vi "EntoLidar_Octoplus.vi"() -> ()   [LabVIEW 2013, in "Octoplus_LIDAR.lvlib"]
uses:
  <userlib>/Octoplus_LIDAR/Octoplus_LIDAR.lvlib
  <vilib>/Analysis/baseanly.llb/Mean (DBL).vi
  <vilib>/Analysis/NI_AALBase.lvlib
  <vilib>/gmath/NI_Gmath.lvlib
panel:
  in  "Boolean":bool
  in  "End 2":dbl min=0.0 max=2047.0 step=1.0
  in  "Start 2":dbl min=0.0 max=2047.0 step=1.0
  out "Meter":dbl(knob) scale=0.0..10.0
  in  "Knob":dbl(knob) scale=0.0..10.0
  in  "End 1":dbl caption="End" min=0.0 max=2047.0 step=1.0
  in  "Start 1":dbl caption="Start" min=0.0 max=2047.0 step=1.0 format="%#_3f"
  in  "Tab Control":T1(tab)
  out "Signal":dbl[][](graph)
  out "Background":dbl[](graph)
  out "XY Graph 2":cluster{"X":dbl, "Y":dbl}[](graph)
  out "XY Graph 3":cluster{"X":dbl, "Y":dbl}[](graph)
  out "XY Graph 2":cluster{"X":dbl, "Y":dbl}[](graph)
  out "Air signal":cluster{timestamp[], dbl[]}(graph)
  out "XY Graph 4":cluster{"X":dbl, "Y":dbl}[](graph)
  in  "Buffer timesout (ms)":u32=30000
  in  "Nbr of lines in Image":u32=6000
  in  "File Path":path=path "C:/Users/USUARIO1/Desktop/Lidar test data"
  in  "Capture":bool
  in  "Record data":bool
  in  "Timeslot (cw, ts1, ts2)":i32(knob)=2 scale=0.0..2.0
  in  "start":bool
  in  "stop":bool
  in  "error in (no error)":errorcluster
  out "error out":errorcluster
  # "ROI 1"
  # "ROI 2"
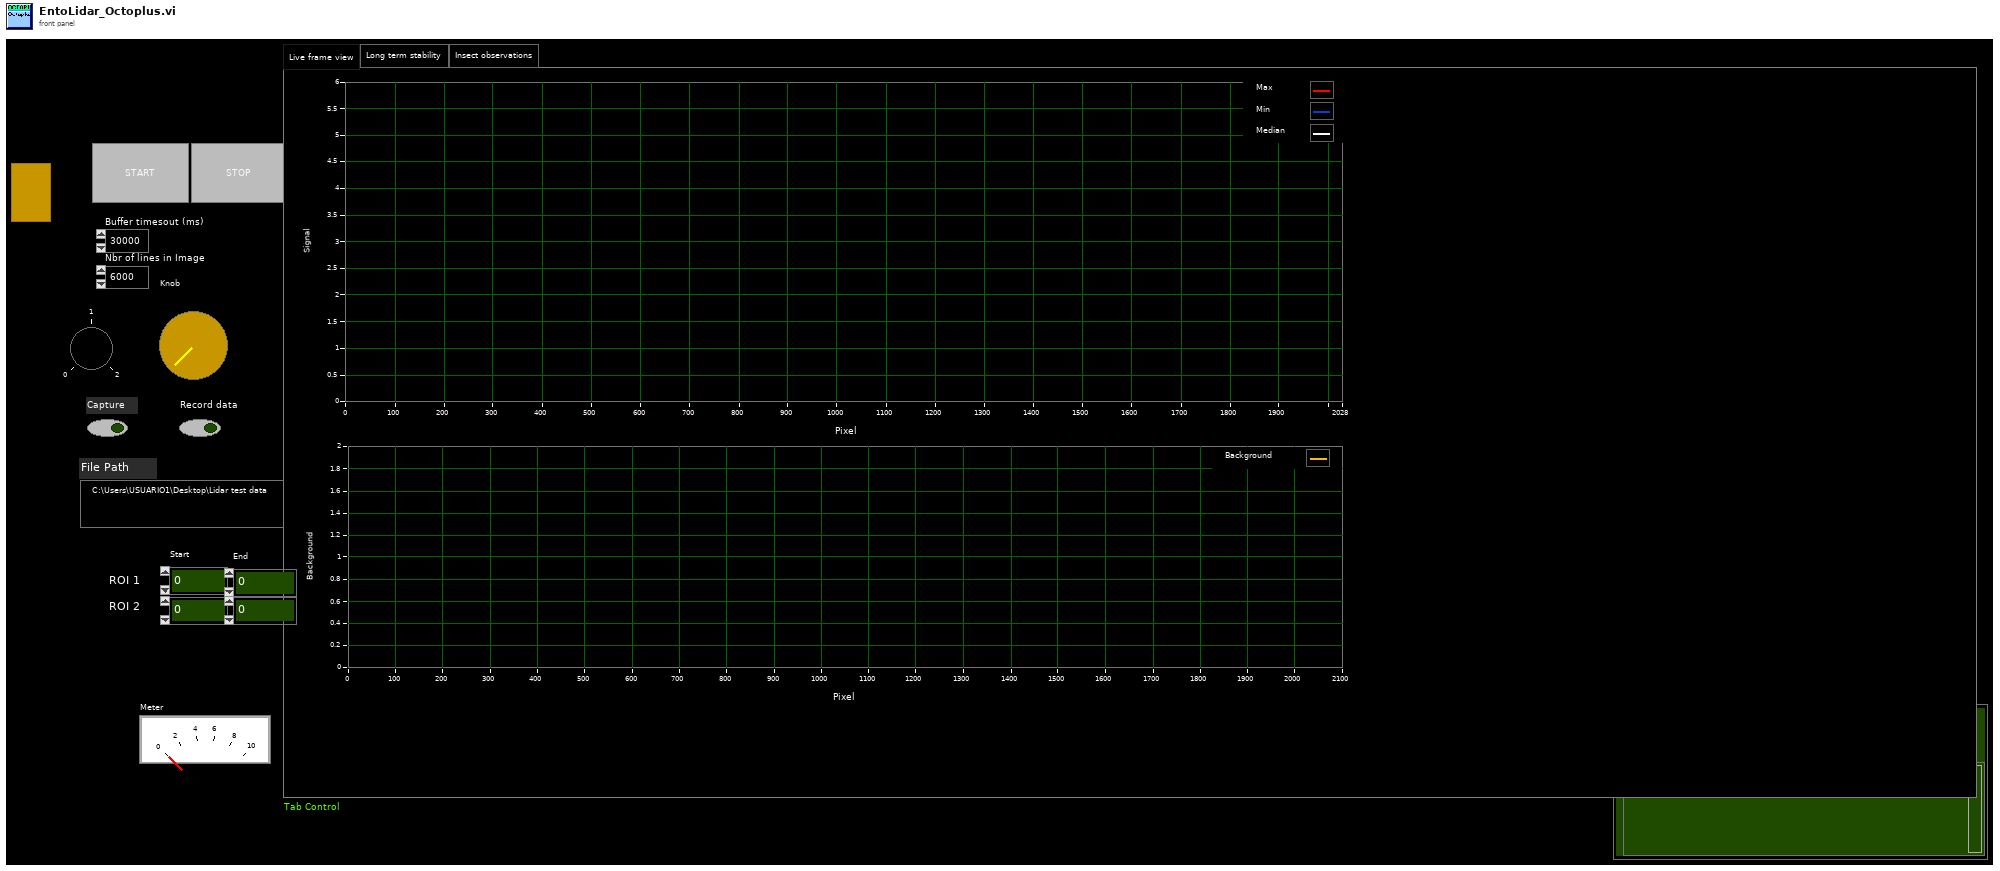
[diagram p1: front panel]
types:
  T1 = enum32{"Live frame view", "Long term stability", "Insect observations"}
  T2 = cluster{"pcID[0]":i8, "pcID[1]":i8, "pcID[2]":i8, "pcID[3]":i8, "pcID[4]":i8, "pcID[5]":i8, "pcID[6]":i8, "pcID[7]":i8, "pcID[8]":i8, "pcID[9]":i8, "pcID[10]":i8, "pcID[11]":i8, "pcID[12]":i8, "pcID[13]":i8, "pcID[14]":i8, "pcID[15]":i8, "pcID[16]":i8, "pcID[17]":i8, "pcID[18]":i8, "pcID[19]":i8, "pcID[20]":i8, "pcID[21]":i8, "pcID[22]":i8, "pcID[23]":i8, "pcID[24]":i8, "pcID[25]":i8, "pcID[26]":i8, "pcID[27]":i8, "pcID[28]":i8, "pcID[29]":i8, "pcID[30]":i8, "pcID[31]":i8, "pcID[32]":i8, "pcID[33]":i8, "pcID[34]":i8, "pcID[35]":i8, "pcID[36]":i8, "pcID[37]":i8, "pcID[38]":i8, "pcID[39]":i8, "pcID[40]":i8, "pcID[41]":i8, "pcID[42]":i8, "pcID[43]":i8, "pcID[44]":i8, "pcID[45]":i8, "pcID[46]":i8, "pcID[47]":i8, "pcID[48]":i8, "pcID[49]":i8, "pcID[50]":i8, "pcID[51]":i8, "pcID[52]":i8, "pcID[53]":i8, "pcID[54]":i8, "pcID[55]":i8, "pcID[56]":i8, "pcID[57]":i8, "pcID[58]":i8, "pcID[59]":i8, "pcID[60]":i8, "pcID[61]":i8, "pcID[62]":i8, "pcID[63]":i8, "pcID[64]":i8, "pcID[65]":i8, "pcID[66]":i8, "pcID[67]":i8, "pcID[68]":i8, "pcID[69]":i8, "pcID[70]":i8, "pcID[71]":i8, "pcID[72]":i8, "pcID[73]":i8, "pcID[74]":i8, "pcID[75]":i8, "pcID[76]":i8, "pcID[77]":i8, "pcID[78]":i8, "pcID[79]":i8, "pcID[80]":i8, "pcID[81]":i8, "pcID[82]":i8, "pcID[83]":i8, "pcID[84]":i8, "pcID[85]":i8, "pcID[86]":i8, "pcID[87]":i8, "pcID[88]":i8, "pcID[89]":i8, "pcID[90]":i8, "pcID[91]":i8, "pcID[92]":i8, "pcID[93]":i8, "pcID[94]":i8, "pcID[95]":i8, "pcID[96]":i8, "pcID[97]":i8, "pcID[98]":i8, "pcID[99]":i8, "pcID[100]":i8, "pcID[101]":i8, "pcID[102]":i8, "pcID[103]":i8, "pcID[104]":i8, "pcID[105]":i8, "pcID[106]":i8, "pcID[107]":i8, "pcID[108]":i8, "pcID[109]":i8, "pcID[110]":i8, "pcID[111]":i8, "pcID[112]":i8, "pcID[113]":i8, "pcID[114]":i8, "pcID[115]":i8, "pcID[116]":i8, "pcID[117]":i8, "pcID[118]":i8, "pcID[119]":i8, "pcID[120]":i8, "pcID[121]":i8, "pcID[122]":i8, "pcID[123]":i8, "pcID[124]":i8, "pcID[125]":i8, "pcID[126]":i8, "pcID[127]":i8, "pcID[128]":i8, "pcID[129]":i8, "pcID[130]":i8, "pcID[131]":i8, "pcID[132]":i8, "pcID[133]":i8, "pcID[134]":i8, "pcID[135]":i8, "pcID[136]":i8, "pcID[137]":i8, "pcID[138]":i8, "pcID[139]":i8, "pcID[140]":i8, "pcID[141]":i8, "pcID[142]":i8, "pcID[143]":i8, "pcID[144]":i8, "pcID[145]":i8, "pcID[146]":i8, "pcID[147]":i8, "pcID[148]":i8, "pcID[149]":i8, "pcID[150]":i8, "pcID[151]":i8, "pcID[152]":i8, "pcID[153]":i8, "pcID[154]":i8, "pcID[155]":i8, "pcID[156]":i8, "pcID[157]":i8, "pcID[158]":i8, "pcID[159]":i8, "pcID[160]":i8, "pcID[161]":i8, "pcID[162]":i8, "pcID[163]":i8, "pcID[164]":i8, "pcID[165]":i8, "pcID[166]":i8, "pcID[167]":i8, "pcID[168]":i8, "pcID[169]":i8, "pcID[170]":i8, "pcID[171]":i8, "pcID[172]":i8, "pcID[173]":i8, "pcID[174]":i8, "pcID[175]":i8, "pcID[176]":i8, "pcID[177]":i8, "pcID[178]":i8, "pcID[179]":i8, "pcID[180]":i8, "pcID[181]":i8, "pcID[182]":i8, "pcID[183]":i8, "pcID[184]":i8, "pcID[185]":i8, "pcID[186]":i8, "pcID[187]":i8, "pcID[188]":i8, "pcID[189]":i8, "pcID[190]":i8, "pcID[191]":i8, "pcID[192]":i8, "pcID[193]":i8, "pcID[194]":i8, "pcID[195]":i8, "pcID[196]":i8, "pcID[197]":i8, "pcID[198]":i8, "pcID[199]":i8, "pcID[200]":i8, "pcID[201]":i8, "pcID[202]":i8, "pcID[203]":i8, "pcID[204]":i8, "pcID[205]":i8, "pcID[206]":i8, "pcID[207]":i8, "pcID[208]":i8, "pcID[209]":i8, "pcID[210]":i8, "pcID[211]":i8, "pcID[212]":i8, "pcID[213]":i8, "pcID[214]":i8, "pcID[215]":i8, "pcID[216]":i8, "pcID[217]":i8, "pcID[218]":i8, "pcID[219]":i8, "pcID[220]":i8, "pcID[221]":i8, "pcID[222]":i8, "pcID[223]":i8, "pcID[224]":i8, "pcID[225]":i8, "pcID[226]":i8, "pcID[227]":i8, "pcID[228]":i8, "pcID[229]":i8, "pcID[230]":i8, "pcID[231]":i8, "pcID[232]":i8, "pcID[233]":i8, "pcID[234]":i8, "pcID[235]":i8, "pcID[236]":i8, "pcID[237]":i8, "pcID[238]":i8, "pcID[239]":i8, "pcID[240]":i8, "pcID[241]":i8, "pcID[242]":i8, "pcID[243]":i8, "pcID[244]":i8, "pcID[245]":i8, "pcID[246]":i8, "pcID[247]":i8, "pcID[248]":i8, "pcID[249]":i8, "pcID[250]":i8, "pcID[251]":i8, "pcID[252]":i8, "pcID[253]":i8, "pcID[254]":i8, "pcID[255]":i8, "pcID[256]":i8, "pcID[257]":i8, "pcID[258]":i8, "pcID[259]":i8}
  T3 = enum16{"open", "replace", "create", "open or create", "replace or create", "replace or create with confirmation"}
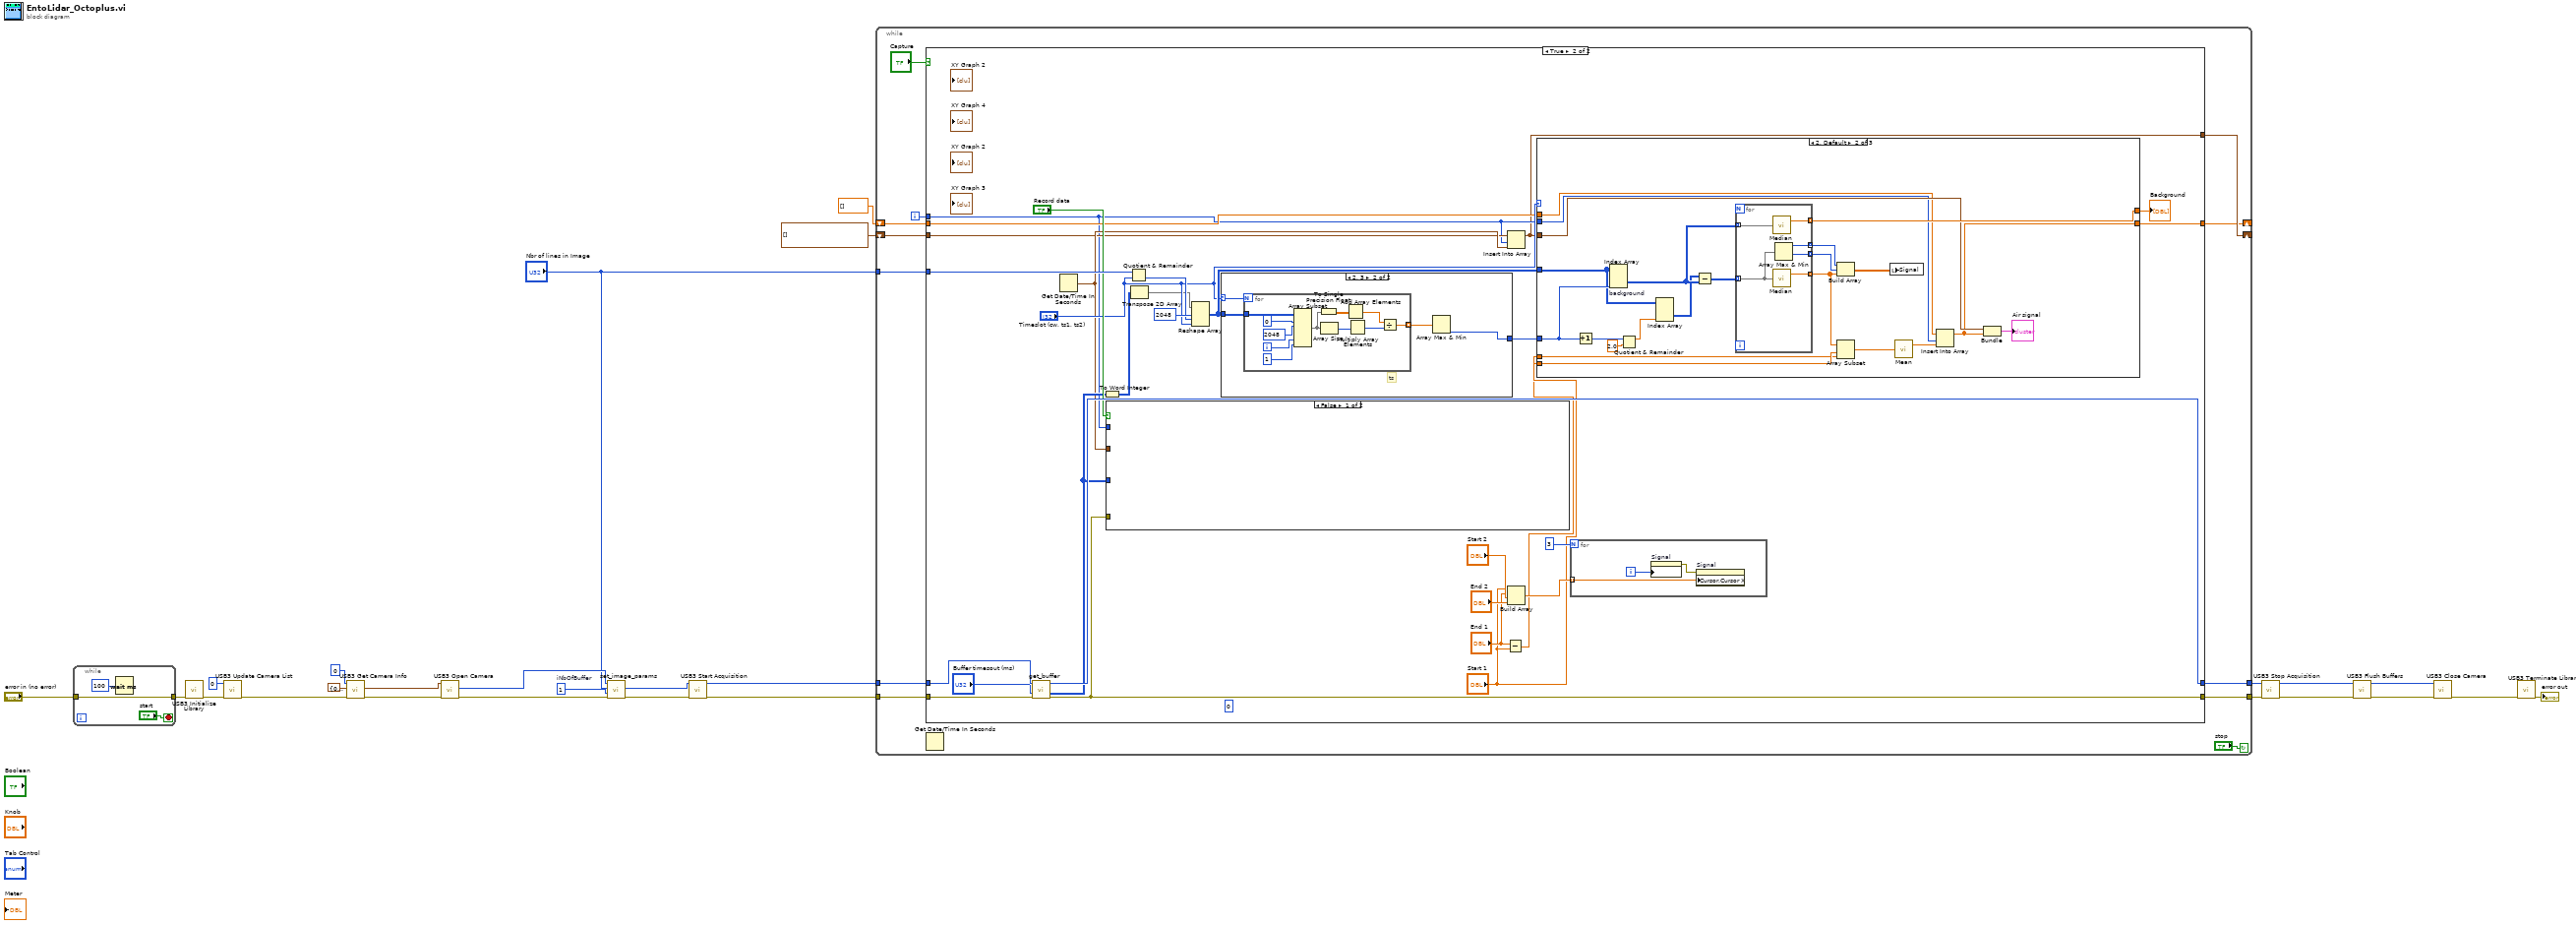
[diagram p0: block diagram]
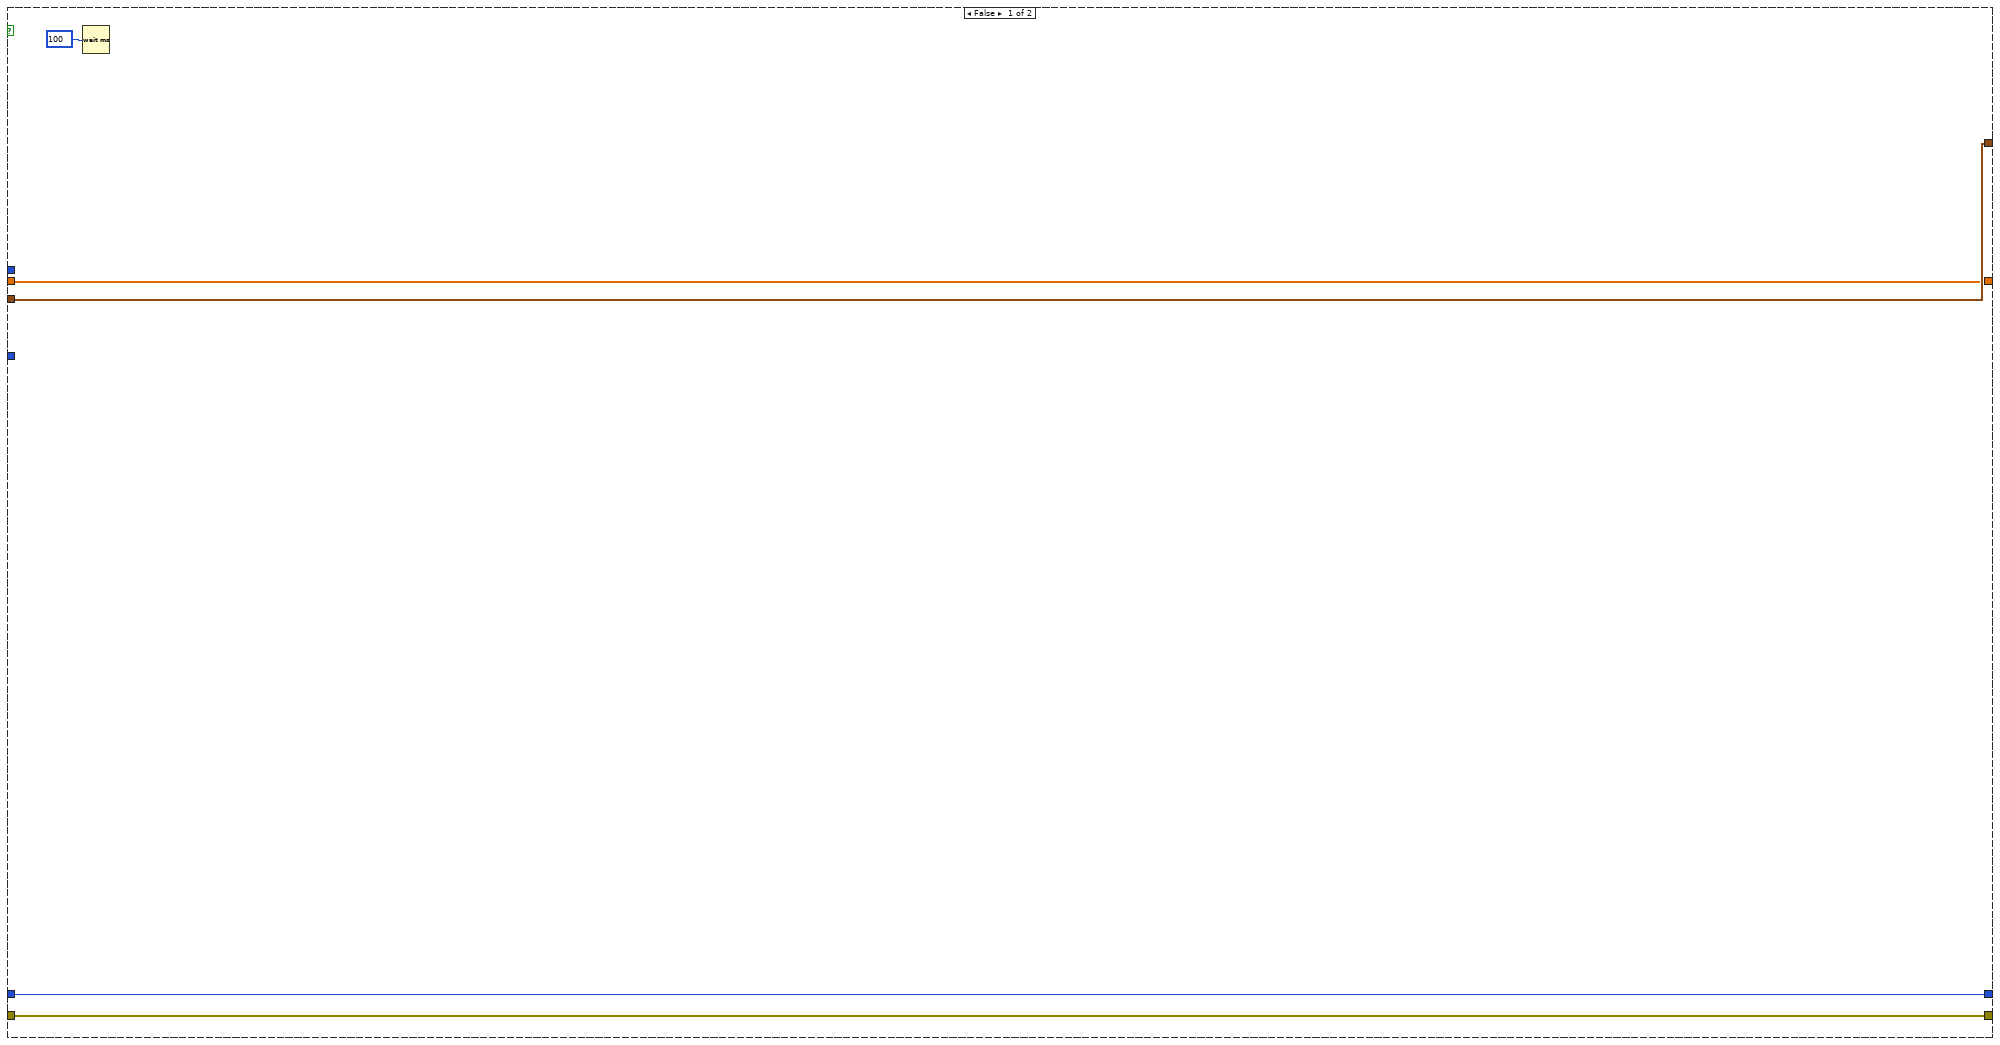
[diagram p2: hidden frame]
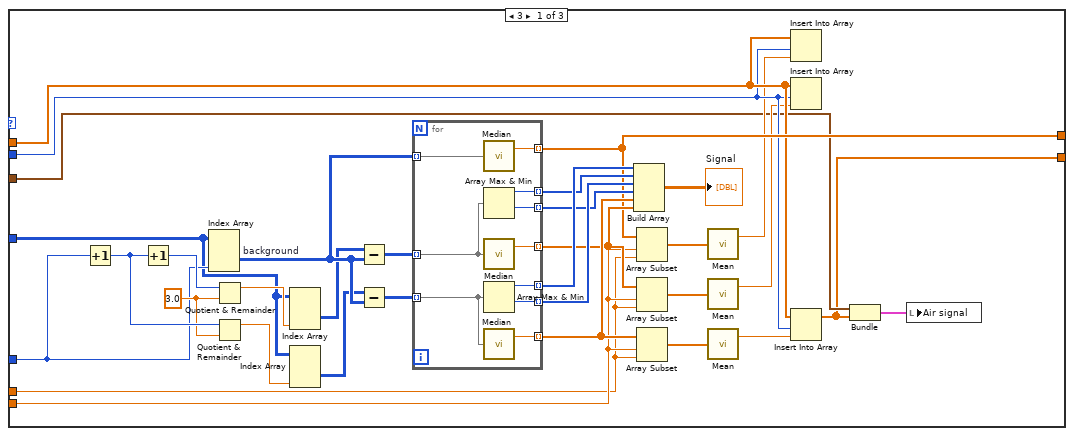
[diagram p3: hidden frame]
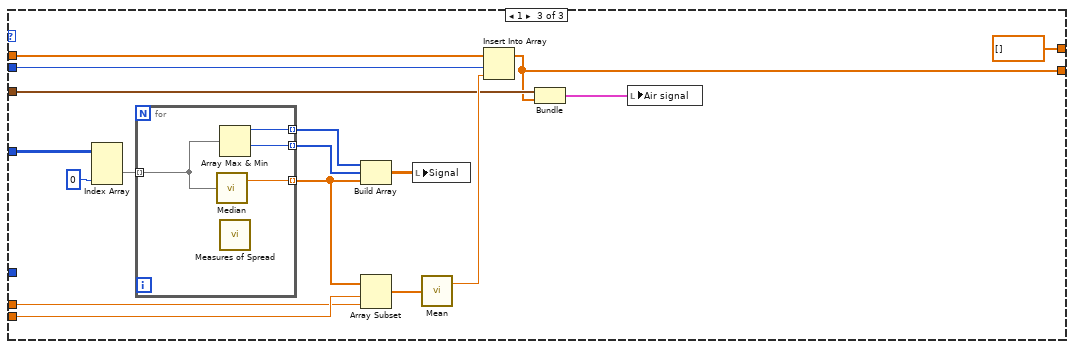
[diagram p4: hidden frame]
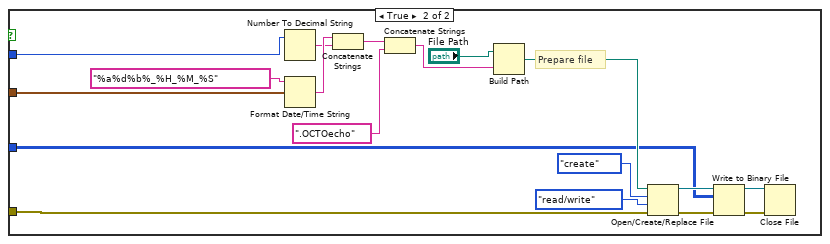
[diagram p5: hidden frame]
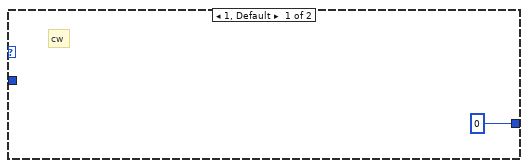
[diagram p6: hidden frame]
diagram:
  w19 = u32 1  # iNbOfBuffer
  n1 = while {
    tunnel: "error in (no error)" -> [w30]
    tunnel: [w30] -> w4
    stop <- "start" stop-if-true
    n2 = Wait (ms)(milliseconds to wait=u32 100) -> ()  [unwired: 1 out]
  }
  n3 = call <userlib>:"USB3 Initialize Library.vi"("error in (no error)"=w4) -> ("error out"=w6:errorcluster)  [unwired: 8 in, 1 out]
  n4 = call <userlib>:"USB3 Update Camera List.vi"("error in (no error)"=w6, "pulNbCameras"=u32 0) -> ("error out"=w24:errorcluster)  [unwired: 7 in, 2 out]
  n5 = call <userlib>:"USB3 Get Camera Info.vi"("error in (no error)"=w24, "pCameraInfo"=T2 {"pcID[0]"=0, "pcID[1]"=0, "pcID[2]"=0, "pcID[3]"=0, "pcID[4]"=0, "pcID[5]"=0, "pcID[6]"=0, "pcID[7]"=0, "pcID[8]"=0, "pcID[9]"=0, "pcID[10]"=0, "pcID[11]"=0, "pcID[12]"=0, "pcID[13]"=0, "pcID[14]"=0, "pcID[15]"=0, "pcID[16]"=0, "pcID[17]"=0, "pcID[18]"=0, "pcID[19]"=0, "pcID[20]"=0, "pcID[21]"=0, "pcID[22]"=0, "pcID[23]"=0, "pcID[24]"=0, "pcID[25]"=0, "pcID[26]"=0, "pcID[27]"=0, "pcID[28]"=0, "pcID[29]"=0, "pcID[30]"=0, "pcID[31]"=0, "pcID[32]"=0, "pcID[33]"=0, "pcID[34]"=0, "pcID[35]"=0, "pcID[36]"=0, "pcID[37]"=0, "pcID[38]"=0, "pcID[39]"=0, "pcID[40]"=0, "pcID[41]"=0, "pcID[42]"=0, "pcID[43]"=0, "pcID[44]"=0, "pcID[45]"=0, "pcID[46]"=0, "pcID[47]"=0, "pcID[48]"=0, "pcID[49]"=0, "pcID[50]"=0, "pcID[51]"=0, "pcID[52]"=0, "pcID[53]"=0, "pcID[54]"=0, "pcID[55]"=0, "pcID[56]"=0, "pcID[57]"=0, "pcID[58]"=0, "pcID[59]"=0, "pcID[60]"=0, "pcID[61]"=0, "pcID[62]"=0, "pcID[63]"=0, "pcID[64]"=0, "pcID[65]"=0, "pcID[66]"=0, "pcID[67]"=0, "pcID[68]"=0, "pcID[69]"=0, "pcID[70]"=0, "pcID[71]"=0, "pcID[72]"=0, "pcID[73]"=0, "pcID[74]"=0, "pcID[75]"=0, "pcID[76]"=0, "pcID[77]"=0, "pcID[78]"=0, "pcID[79]"=0, "pcID[80]"=0, "pcID[81]"=0, "pcID[82]"=0, "pcID[83]"=0, "pcID[84]"=0, "pcID[85]"=0, "pcID[86]"=0, "pcID[87]"=0, "pcID[88]"=0, "pcID[89]"=0, "pcID[90]"=0, "pcID[91]"=0, "pcID[92]"=0, "pcID[93]"=0, "pcID[94]"=0, "pcID[95]"=0, "pcID[96]"=0, "pcID[97]"=0, "pcID[98]"=0, "pcID[99]"=0, "pcID[100]"=0, "pcID[101]"=0, "pcID[102]"=0, "pcID[103]"=0, "pcID[104]"=0, "pcID[105]"=0, "pcID[106]"=0, "pcID[107]"=0, "pcID[108]"=0, "pcID[109]"=0, "pcID[110]"=0, "pcID[111]"=0, "pcID[112]"=0, "pcID[113]"=0, "pcID[114]"=0, "pcID[115]"=0, "pcID[116]"=0, "pcID[117]"=0, "pcID[118]"=0, "pcID[119]"=0, "pcID[120]"=0, "pcID[121]"=0, "pcID[122]"=0, "pcID[123]"=0, "pcID[124]"=0, "pcID[125]"=0, "pcID[126]"=0, "pcID[127]"=0, "pcID[128]"=0, "pcID[129]"=0, "pcID[130]"=0, "pcID[131]"=0, "pcID[132]"=0, "pcID[133]"=0, "pcID[134]"=0, "pcID[135]"=0, "pcID[136]"=0, "pcID[137]"=0, "pcID[138]"=0, "pcID[139]"=0, "pcID[140]"=0, "pcID[141]"=0, "pcID[142]"=0, "pcID[143]"=0, "pcID[144]"=0, "pcID[145]"=0, "pcID[146]"=0, "pcID[147]"=0, "pcID[148]"=0, "pcID[149]"=0, "pcID[150]"=0, "pcID[151]"=0, "pcID[152]"=0, "pcID[153]"=0, "pcID[154]"=0, "pcID[155]"=0, "pcID[156]"=0, "pcID[157]"=0, "pcID[158]"=0, "pcID[159]"=0, "pcID[160]"=0, "pcID[161]"=0, "pcID[162]"=0, "pcID[163]"=0, "pcID[164]"=0, "pcID[165]"=0, "pcID[166]"=0, "pcID[167]"=0, "pcID[168]"=0, "pcID[169]"=0, "pcID[170]"=0, "pcID[171]"=0, "pcID[172]"=0, "pcID[173]"=0, "pcID[174]"=0, "pcID[175]"=0, "pcID[176]"=0, "pcID[177]"=0, "pcID[178]"=0, "pcID[179]"=0, "pcID[180]"=0, "pcID[181]"=0, "pcID[182]"=0, "pcID[183]"=0, "pcID[184]"=0, "pcID[185]"=0, "pcID[186]"=0, "pcID[187]"=0, "pcID[188]"=0, "pcID[189]"=0, "pcID[190]"=0, "pcID[191]"=0, "pcID[192]"=0, "pcID[193]"=0, "pcID[194]"=0, "pcID[195]"=0, "pcID[196]"=0, "pcID[197]"=0, "pcID[198]"=0, "pcID[199]"=0, "pcID[200]"=0, "pcID[201]"=0, "pcID[202]"=0, "pcID[203]"=0, "pcID[204]"=0, "pcID[205]"=0, "pcID[206]"=0, "pcID[207]"=0, "pcID[208]"=0, "pcID[209]"=0, "pcID[210]"=0, "pcID[211]"=0, "pcID[212]"=0, "pcID[213]"=0, "pcID[214]"=0, "pcID[215]"=0, "pcID[216]"=0, "pcID[217]"=0, "pcID[218]"=0, "pcID[219]"=0, "pcID[220]"=0, "pcID[221]"=0, "pcID[222]"=0, "pcID[223]"=0, "pcID[224]"=0, "pcID[225]"=0, "pcID[226]"=0, "pcID[227]"=0, "pcID[228]"=0, "pcID[229]"=0, "pcID[230]"=0, "pcID[231]"=0, "pcID[232]"=0, "pcID[233]"=0, "pcID[234]"=0, "pcID[235]"=0, "pcID[236]"=0, "pcID[237]"=0, "pcID[238]"=0, "pcID[239]"=0, "pcID[240]"=0, "pcID[241]"=0, "pcID[242]"=0, "pcID[243]"=0, "pcID[244]"=0, "pcID[245]"=0, "pcID[246]"=0, "pcID[247]"=0, "pcID[248]"=0, "pcID[249]"=0, "pcID[250]"=0, "pcID[251]"=0, "pcID[252]"=0, "pcID[253]"=0, "pcID[254]"=0, "pcID[255]"=0, "pcID[256]"=0, "pcID[257]"=0, "pcID[258]"=0, "pcID[259]"=0}, "ulIndex"=u32 0) -> ("error out"=w22:errorcluster, "pCameraInfo out"=w23:T2)  [unwired: 6 in, 1 out]
  n6 = call <userlib>:"USB3 Open Camera.vi"("error in (no error)"=w22, "pCameraInfo"=w23) -> ("error out"=w21:errorcluster, "hCamera"=w20:u64)  [unwired: 7 in, 1 out]
  n7 = call <userlib>:"set_image_params.vi"("error in (no error)"=w21, "iNbOfBuffer"=w19, "iImageHeight"="Nbr of lines in Image", "hCamera"=w20) -> ("error out"=w18:errorcluster, "hCamera"=w9:u64)  [unwired: 5 in, 1 out]
  n8 = call <userlib>:"USB3 Start Acquisition.vi"("error in (no error)"=w18, "hCamera"=w9) -> ("error out"=w16:errorcluster, "hCamera"=w17:u64)  [unwired: 7 in, 1 out]
  n9 = while {
    tunnel: w17 -> [w42]
    tunnel: w16 -> [w41]
    tunnel: [w38] -> w15
    tunnel: [w40] -> w12
    tunnel: "Nbr of lines in Image" -> [w36]
    shift-right: [w34] -> _
    shift-left: timestamp[] [] -> [w33]
    shift-right: [w32] -> _
    shift-left: dbl[] [] -> [w31]
    i -> [w35]
    stop <- "stop" continue-if-true
    n10 = case shown="True" "Capture" {
      tunnel: w42 -> [w45 w76]
      tunnel: w41 -> [w46 w75]
      tunnel: [w45 w74] -> w40
      tunnel: [w46 w67] -> w38
      tunnel: w36 -> [_ w70]
      tunnel: w35 -> [_ w50]
      tunnel: [w44 w49] -> w34
      tunnel: w33 -> [w44 w55]
      tunnel: w31 -> [w43 w51]
      tunnel: [w43 w48] -> w32
      frame False {
        n11 = Wait (ms)(milliseconds to wait=u32 100) -> ()  [unwired: 1 out]
      }
      frame True {
        (unwired) 0 ("index")
        n12 = call <userlib>:"get_buffer.vi"("error in (no error)"=w75, "ulTimeoutInMs"="Buffer timesout (ms)", "hCamera"=w76) -> ("error out"=w67:errorcluster, "output array"=w61:u16[][], "hCamera out"=w74:u64)  [unwired: 5 in, 1 out]
        n13 = Get Date/Time In Seconds() -> (seconds since 1Jan1904=w56:timestamp)
        n14 = To Word Integer(number=w61) -> (16bit integer=w62:i16[][])
        n15 = case shown="False" "Record data" {
          tunnel: w67 -> [_ w182]
          tunnel: w61 -> [_ w177]
          tunnel: w50 -> [_ w173]
          tunnel: w56 -> [_ w172]
          frame False {
          }
          frame True {
            # "Prepare file"
            n16 = Number To Decimal String(number=w173) -> (decimal integer string=w174:string)  [unwired: 1 in]
            n17 = Format Date/Time String(time format string (%c)="%a%d%b%_%H_%M_%S", seconds (now)=w172) -> (date/time string=w175:string)  [unwired: 1 in]
            n18 = Concatenate Strings(w175, w174) -> (w176:string)
            n19 = Concatenate Strings(w176, ".OCTOecho") -> (w179:string)
            n20 = Build Path(base path="File Path", name or relative path=w179) -> (appended path=w181:path)
            n21 = Open/Create/Replace File(file path (use dialog)=w181, error in=w182, operation (0:open)=T3."create", access (0:read/write)=enum16{"read/write", "read-only", "write-only"}."read/write") -> (refnum out=w187:refnum<file>, error out=w183:errorcluster)  [unwired: 3 out]
            n22 = Write to Binary File(file (use dialog)=w187, data=w177, error in=w183) -> (refnum out=w185:refnum<file>, error out=w184:errorcluster)  [unwired: 1 in, 3 out]
            n23 = Close File(refnum=w185, error in=w184) -> ()  [unwired: 2 out]
          }
        }
        n24 = Quotient & Remainder(x=w70, y="Timeslot (cw, ts1, ts2)") -> (floor(x/y)=w69:u32)  [unwired: 1 out]
        n25 = Transpose 2D Array(2D array=w62) -> (transposed array=w63:i16[][])
        n26 = Reshape Array(w63, 2048 ("dimension size"), w69, "Timeslot (cw, ts1, ts2)") -> (w65:i16[][][])
        n27 = case shown="2, 3" "Timeslot (cw, ts1, ts2)" {
          selector: "Timeslot (cw, ts1, ts2)" -> [_ w191]
          tunnel: [0 w193] -> w66
          tunnel: w65 -> [_ w192]
          frame 1, Default {
            # "cw"
          }
          frame 2, 3 {
            # "ts"
            n28 = for {
              N: w191 -> [_]
              tunnel: [w204] -> w194 mode=indexing
              tunnel: w192 -> [w199]
              i -> [w201]
              n29 = Array Subset(array=w199, index (dim 0)=0 ("index"), length (dim 0)=2048 ("length"), index (dim 2)=w201, length (dim 2)=1 ("intervals")) -> (w196:i16[][][])  [unwired: 2 in]
              n30 = To Single Precision Float(number=w196) -> (single precision float=w195:sgl[][][])
              n31 = Array Size(array=w196) -> (size(s)=w202:i32[])
              n32 = Add Array Elements(numeric array=w195) -> (sum=w203:sgl)
              n33 = Multiply Array Elements(1:w202) -> (0:w205:i32)
              n34 = Divide(x=w203, y=w205) -> (x/y=w204:sgl)
            }
            n35 = Array Max & Min(array=w194) -> (min index (indices)=w193:i32)  [unwired: 3 out]
          }
        }
        n36 = Subtract(x="End 1", y="Start 1") -> (x-y=w52:dbl)
        n37 = Insert Into Array(array=w55, index=w50, new element=w56) -> (w49:timestamp[])
        n38 = Build Array("Start 1", "End 1", "Start 2", "End 2") -> (w57:dbl[])
        n39 = case shown="2, Default" "Timeslot (cw, ts1, ts2)" {
          tunnel: [w90 w144 dbl[] []] -> w72
          tunnel: w66 -> [w109 w141 _]
          tunnel: w65 -> [w106 w139 w167]
          tunnel: "Start 1" -> [w89 w125 w159]
          tunnel: w52 -> [w88 w124 w158]
          tunnel: w51 -> [w87 w127 w154]
          tunnel: w50 -> [w86 w126 w155]
          tunnel: w49 -> [w82 w128 w153]
          tunnel: [w80 w123 w152] -> w48
          frame 3 {
            w111 = 3.0 ("y")
            n40 = Increment(x=w109) -> (x+1=w112:i32)
            n41 = Increment(x=w112) -> (x+1=w110:i32)
            n42 = Index Array "background"(array=w106, index (dim 2)=w109) -> (element=w105:i16[][])  [unwired: 2 in]
            n43 = Quotient & Remainder(x=w110, y=w111) -> (x-y*floor(x/y)=w107:dbl)  [unwired: 1 out]
            n44 = Quotient & Remainder(x=w112, y=w111) -> (x-y*floor(x/y)=w108:dbl)  [unwired: 1 out]
            n45 = Index Array(array=w106, index (dim 2)=w107) -> (element=w104:i16[][])  [unwired: 2 in]
            n46 = Index Array(array=w106, index (dim 2)=w108) -> (element=w101:i16[][])  [unwired: 2 in]
            n47 = Subtract(x=w104, y=w105) -> (x-y=w102:i16[][])
            n48 = Subtract(x=w101, y=w105) -> (x-y=w103:i16[][])
            n49 = for {
              tunnel: [w122] -> w95 mode=indexing
              tunnel: [w121] -> w98 mode=indexing
              tunnel: [w120] -> w100 mode=indexing
              tunnel: [w119] -> w90 mode=indexing
              tunnel: w105 -> [w118] mode=indexing
              tunnel: w103 -> [w117] mode=indexing
              tunnel: w102 -> [w116] mode=indexing
              tunnel: [w115] -> w99 mode=indexing
              tunnel: [w114] -> w97 mode=indexing
              tunnel: [w113] -> w91 mode=indexing
              n50 = call <vilib>:"Median.vi"("X"=w118) -> ("median"=w119:dbl)  [unwired: 1 out]
              n51 = Array Max & Min(array=w116) -> (max value=w115:i16, min value=w114:i16)  [unwired: 2 out]
              n52 = call <vilib>:"Median.vi"("X"=w116) -> ("median"=w113:dbl)  [unwired: 1 out]
              n53 = Array Max & Min(array=w117) -> (max value=w120:i16, min value=w121:i16)  [unwired: 2 out]
              n54 = call <vilib>:"Median.vi"("X"=w117) -> ("median"=w122:dbl)  [unwired: 1 out]
            }
            n55 = Build Array(w100, w99, w98, w97, w95, w91) -> (→"Signal":dbl[][])
            n56 = Array Subset(array=w90, index=w89, length=w88) -> (w92:dbl[])
            n57 = Array Subset(array=w91, index=w89, length=w88) -> (w93:dbl[])
            n58 = Array Subset(array=w95, index=w89, length=w88) -> (w94:dbl[])
            n59 = call-poly <vilib>:"Mean.vi"("X"=w92) -> ("mean"=w85:dbl)  [unwired: 1 out]
            n60 = call-poly <vilib>:"Mean.vi"("X"=w93) -> ("mean"=w84:dbl)  [unwired: 1 out]
            n61 = call-poly <vilib>:"Mean.vi"("X"=w94) -> ("mean"=w83:dbl)  [unwired: 1 out]
            n62 = Insert Into Array(array=w87, index=w86, new element=w85) -> ()  [unwired: 1 out]
            n63 = Insert Into Array(array=w87, index=w86, new element=w84) -> ()  [unwired: 1 out]
            n64 = Insert Into Array(array=w87, index=w86, new element=w83) -> (w80:dbl[])
            n65 = Bundle(w82, w80) -> (w81:cluster{timestamp[], dbl[]})  [unwired: 1 in]
            n66 = local write "Air signal"(w81) -> ()
          }
          frame 2, Default {
            n67 = Increment(x=w141) -> (x+1=w143:i32)
            n68 = Index Array "background"(array=w139, index (dim 2)=w141) -> (element=w138:i16[][])  [unwired: 2 in]
            n69 = Quotient & Remainder(x=w143, y=2.0) -> (x-y*floor(x/y)=w140:dbl)  [unwired: 1 out]
            n70 = Index Array(array=w139, index (dim 2)=w140) -> (element=w136:i16[][])  [unwired: 2 in]
            n71 = Subtract(x=w136, y=w138) -> (x-y=w137:i16[][])
            n72 = for {
              tunnel: [w150] -> w132 mode=indexing
              tunnel: [w149] -> w134 mode=indexing
              tunnel: [w148] -> w135 mode=indexing
              tunnel: [w147] -> w144 mode=indexing
              tunnel: w138 -> [w146] mode=indexing
              tunnel: w137 -> [w145] mode=indexing
              n73 = call <vilib>:"Median.vi"("X"=w146) -> ("median"=w147:dbl)  [unwired: 1 out]
              n74 = call <vilib>:"Median.vi"("X"=w145) -> ("median"=w150:dbl)  [unwired: 1 out]
              n75 = Array Max & Min(array=w145) -> (max value=w148:i16, min value=w149:i16)  [unwired: 2 out]
            }
            n76 = Build Array(w135, w134, w132) -> (w133:dbl[][])
            n77 = Array Subset(array=w132, index=w125, length=w124) -> (w131:dbl[])
            n78 = local write "Signal"(w133) -> ()
            n79 = call-poly <vilib>:"Mean.vi"("X"=w131) -> ("mean"=w130:dbl)  [unwired: 1 out]
            n80 = Insert Into Array(array=w127, index=w126, new element=w130) -> (w123:dbl[])
            n81 = Bundle(w128, w123) -> (→"Air signal":cluster{timestamp[], dbl[]})  [unwired: 1 in]
          }
          frame 1 {
            n82 = Index Array(array=w167, index (dim 2)=0 ("index (col)")) -> (element=w165:i16[][])  [unwired: 2 in]
            n83 = for {
              tunnel: [w171] -> w160 mode=indexing
              tunnel: [w170] -> w162 mode=indexing
              tunnel: [w168] -> w163 mode=indexing
              tunnel: w165 -> [w169] mode=indexing
              n84 = call <vilib>:"Median.vi"("X"=w169) -> ("median"=w171:dbl)  [unwired: 1 out]
              n85 = Array Max & Min(array=w169) -> (max value=w168:i16, min value=w170:i16)  [unwired: 2 out]
              n86 = call <vilib>:"Measures of Spread.vi"() -> ()  [unwired: 10 in, 2 out]
            }
            n87 = Build Array(w163, w162, w160) -> (w161:dbl[][])
            n88 = Array Subset(array=w160, index=w159, length=w158) -> (w157:dbl[])
            n89 = local write "Signal"(w161) -> ()
            n90 = call-poly <vilib>:"Mean.vi"("X"=w157) -> ("mean"=w156:dbl)  [unwired: 1 out]
            n91 = Insert Into Array(array=w154, index=w155, new element=w156) -> (w152:dbl[])
            n92 = Bundle(w153, w152) -> (w151:cluster{timestamp[], dbl[]})  [unwired: 1 in]
            n93 = local write "Air signal"(w151) -> ()
          }
        }
        "Background" <- w72
        n94 = for {
          N: 3 -> [_]
          tunnel: w57 -> [w79] mode=indexing
          i -> [w78]
          n95 = property on="Signal" class="WFGraph (strict)"("Active Cursor"=w78) -> (error out=w77:errorcluster)  [unwired: 2 in, 1 out]
          n96 = property on="Signal" class="WFGraph (strict)"(error in=w77, "Cursor.Cursor X"=w79) -> ()  [unwired: 1 in, 2 out]
        }
      }
    }
    n97 = Get Date/Time In Seconds() -> ()  [unwired: 1 out]
  }
  n98 = call <userlib>:"USB3 Stop Acquisition.vi"("error in (no error)"=w15, "hCamera"=w12) -> ("error out"=w14:errorcluster, "hCamera out"=w11:u64)  [unwired: 7 in, 1 out]
  n99 = call <userlib>:"USB3 Flush Buffers.vi"("error in (no error)"=w14, "hCamera"=w11) -> ("error out"=w13:errorcluster, "hCamera out"=w10:u64)  [unwired: 7 in, 1 out]
  n100 = call <userlib>:"USB3 Close Camera.vi"("error in (no error)"=w13, "hCamera"=w10) -> ("error out"=w8:errorcluster)  [unwired: 7 in, 2 out]
  n101 = call <userlib>:"USB3 Terminate Library.vi"("error in (no error)"=w8) -> ("error out"=→"error out":errorcluster)  [unwired: 9 in, 1 out]
